vi "2_2_VisualAD_Inference(Camera).vi"() -> ()   [LabVIEW 2020]
uses:
  <vilib>/Ngene/DeepLTK Anomaly Detection Addon/Toolkit/API/Controls/NN_Paths.ctl
  <vilib>/Ngene/Deep Learning Toolkit/Toolkit/NN_Data/API/NN_Dims(C,H,W).ctl
  <vilib>/Ngene/Deep Learning Toolkit/Toolkit/NN_Network/Controls/NN_Device.ctl
  subVIs/Visualizer/Controls/Display_Options.ctl
  subVIs/Visualizer/Controls/ROI_Display_Options.ctl
  subVIs/Visualizer/Controls/Heatmap_Display_Options.ctl
  subVIs/Visualizer/Controls/ColorMap.ctl
  <vilib>/Ngene/DeepLTK Anomaly Detection Addon/Toolkit/API/Controls/MinMax.ctl
  subVIs/Visualizer/Controls/Report_Images_CFG.ctl
  subVIs/Camera/Controls/Camera_Settings.ctl
  <vilib>/Ngene/DeepLTK Anomaly Detection Addon/Toolkit/API/Controls/Crop_CFG.ctl
  <vilib>/Ngene/DeepLTK Anomaly Detection Addon/Toolkit/API/Controls/NNPC_Setup.ctl
  <vilib>/vision/driver/IMAQdx.llb/IMAQdx Camera Control Mode.ctl
  <vilib>/vision/driver/IMAQdx.llb/IMAQdx Buffer Number Mode.ctl
  <vilib>/Ngene/DeepLTK Anomaly Detection Addon/Toolkit/API/Controls/Feature_Scorer_Params.ctl
  <vilib>/Ngene/DeepLTK Anomaly Detection Addon/Toolkit/API/Controls/Gaussian_Blur.ctl
  <vilib>/Ngene/DeepLTK Anomaly Detection Addon/Toolkit/API/NNPC_Predict/NNPC_Predict(Single).vi
  <vilib>/Ngene/DeepLTK Anomaly Detection Addon/Toolkit/DeepLTK_Anomaly_Detection_Addon.lvlib
  <vilib>/ptbypt/NI_PtbyPt.lvlib
  <vilib>/vision/driver/NI_Vision_Acquisition_Software.lvlib
  <vilib>/Ngene/Deep Learning Toolkit/Toolkit/Deep_Learning_Toolkit_by_Ngene.lvlib
  <vilib>/Ngene/CuLab - GPU Accelerated Toolkit/Toolkit/CuLab.lvlib
panel:
  in  "Crop_CFG":T1={"Left"=0.0, "Top"=0.0, "Right"=1.0, "Bottom"=1.0}
  in  "Camera_Settings":T2={"Camera_Resolution"=10, "Focus"=0, "Exposure"=5, "Gain"=1, "WhiteB."=3000} {"WhiteB." min=2000 max=7500 step=1; "Gain" max=255 step=5; "Exposure" min=0 max=9 step=5; "Focus" step=5}
  in  "Rel Margin":sgl=0.02
  in  "Camera":refnum<k21>="cam0" caption="IMAQdx Session"
  out "Device Name":string="NVIDIA GeForce GTX 1650 Ti"
  in  "Display_Options":T3={"ROI_Options"={"Color"=16711713, "Width"=4, "Drawing Mode"=enum."Frame"}, "Heatmap_Options"={"ColorMap"=enum."Jet", "Alpha"=0.4, "Heatmap Range"={"Min"=25.0, "Max"=32.0}}, "Report_Images_CFG"={"Original Image"=TRUE, "Ground Truth"=TRUE, "HeatMap"=TRUE, "Mask"=TRUE, "Segmentation"=TRUE}} {"Heatmap_Options"."Heatmap Range"."Min" format="%#_5g"}
  in  "Trained_Model_Paths":T9={"CFG"=path "D:/Ngene/GitHub/deepltk_examples/3_Image_Processing/36_Anomaly_Detection/Models/NNPC_Cards_3ofHearts__25_10_21__19_21_13/NNPC_Cards_3ofHearts_25_10_21__19_21_13.cfg", "BIN"=path "D:/Ngene/GitHub/deepltk_examples/3_Image_Processing/36_Anomaly_Detection/Models/NNPC_Cards_3ofHearts__25_10_21__19_21_13/NNPC_Cards_3ofHearts_25_10_21__19_21_13.bin"}
  out "Anomaly?":bool=TRUE
  in  "Device":T10=enum."GPU"
  out "Dims_In":T11={"C"=3, "H"=120, "W"=160}
  out "Loop Time":dbl=0.02274215600000389 format="%.2ps"
  out "Preproc. Time":dbl=0.0010668470000018714 format="%.2ps"
  in  "Image_Thrshld":sgl=-1.0 format="%_5g"
  out "Pixel_Score(Max)":sgl=48.99041
  out "Img_Score":sgl=51.375824
  in  "Pixel_Thrshld":sgl=28.1 format="%_5g"
  out "Inference Time":dbl=0.010325968000006468 format="%.2ps"
  in  "Stop":bool
  out "Anomaly Detection Results":T12(plugin-control)
  # "Unsupervised \nVisual Anomaly Detection"
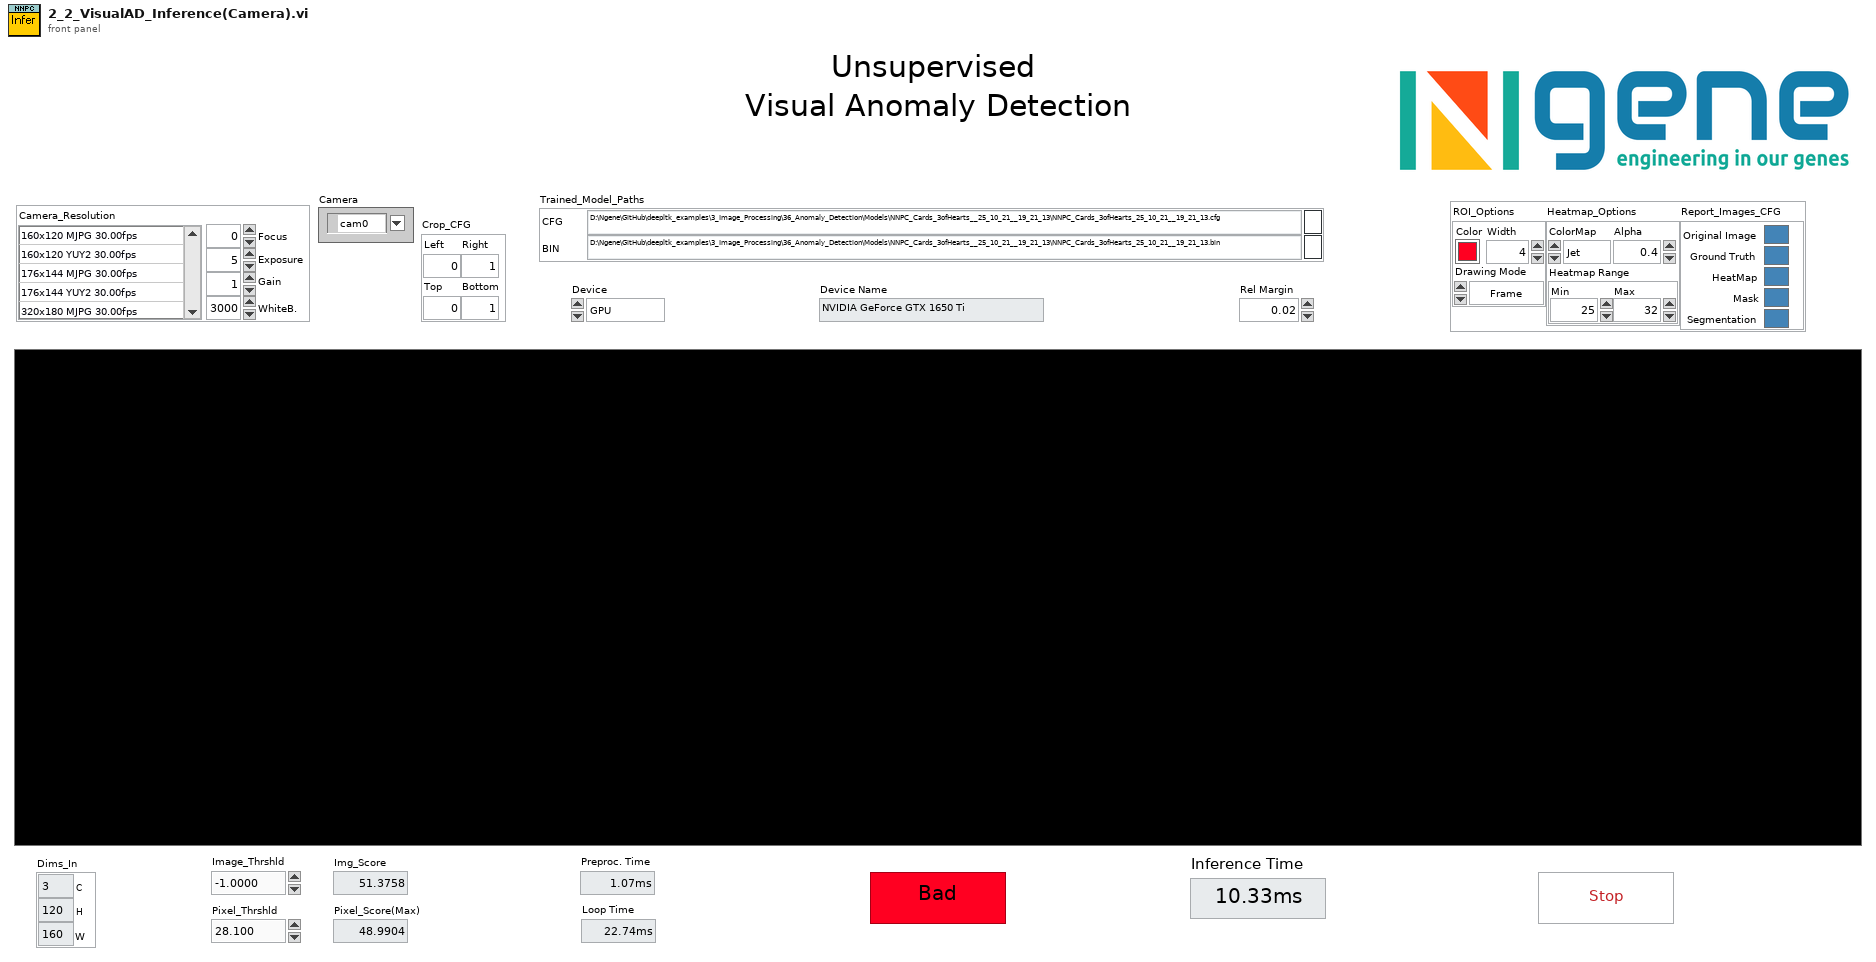
[diagram p1: front panel]
types:
  T1 = typedef "DeepLTK_Anomaly_Detection_Addon.lvlib/Crop_CFG.ctl" = cluster{"Left":sgl, "Top":sgl, "Right":sgl, "Bottom":sgl}
  T2 = typedef "Camera_Settings.ctl" = cluster{"Camera_Resolution":i32, "Focus":u8, "Exposure":i32, "Gain":u32, "WhiteB.":i32}
  T3 = typedef "Display_Options.ctl" = cluster{"ROI_Options":T4, "Heatmap_Options":T5, "Report_Images_CFG":T8}
  T4 = typedef "ROI_Display_Options.ctl" = cluster{"Color":u32, "Width":u32, "Drawing Mode":enum16{"Frame", "Fill"}}
  T5 = typedef "Heatmap_Display_Options.ctl" = cluster{"ColorMap":T6, "Alpha":sgl, "Heatmap Range":T7}
  T6 = typedef "ColorMap.ctl" = enum16{"Jet", "Perula", "Inferno", "Plasma", "Viridis"}
  T7 = typedef "DeepLTK_Anomaly_Detection_Addon.lvlib/MinMax.ctl" = cluster{"Min":sgl, "Max":sgl}
  T8 = typedef "Report_Images_CFG.ctl" = cluster{"Original Image":bool, "Ground Truth":bool, "HeatMap":bool, "Mask":bool, "Segmentation":bool}
  T9 = typedef "DeepLTK_Anomaly_Detection_Addon.lvlib/NN_Paths.ctl" = cluster{"CFG":path, "BIN":path}
  T10 = typedef "Deep_Learning_Toolkit_by_Ngene.lvlib/NN_Device.ctl" = enum16{"CPU", "GPU"}
  T11 = typedef "Deep_Learning_Toolkit_by_Ngene.lvlib/NN_Dims(C,H,W).ctl" = cluster{"C":i32, "H":i32, "W":i32}
  T12 = typedef "IMAQ Image.ctl" = refnum<image>
  T13 = typedef "NI_Vision_Acquisition_Software.lvlib/IMAQdx Camera Control Mode.ctl" = enum32{"Controller", "Listener"}
  T14 = typedef "Image Type" = u32
  T15 = typedef "DeepLTK_Anomaly_Detection_Addon.lvlib/NNPC_Setup.ctl" = cluster{"Input_Dims":T11, "mBatch":i32, "Device":T10, "GPU Id":i32}
  T16 = typedef "IMAQdx.ctl" = refnum<k21>
  T17 = typedef "DeepLTK_Anomaly_Detection_Addon.lvlib/NNPC_Evaluation_Results.ctl" = cluster{"Threshold(Image)":sgl, "Threshold(Pixel)":sgl, "Pixel_Range":cluster{"Min":sgl, "Max":sgl}}
  T18 = typedef "DeepLTK_Anomaly_Detection_Addon.lvlib/NNPC_PreProcessing_Options.ctl" = cluster{"DS_Name":string, "Input_Dims":T11, "Cropping":T1, "Interpolation Type":u32, "MultiStage_ReSample?":bool, "Dataset_Stats":T19}
  T19 = typedef "DeepLTK_Anomaly_Detection_Addon.lvlib/NNPC_DS_Stats.ctl" = cluster{"means":T20, "stds":T20}
  T20 = typedef "DeepLTK_Anomaly_Detection_Addon.lvlib/Image_Stats_RGB.ctl" = cluster{"R":sgl, "G":sgl, "B":sgl}
  T21 = typedef "DeepLTK_Anomaly_Detection_Addon.lvlib/NNPC_Instance.ctl" = cluster{"Name":string, "NN":T22, "MemBank_Data":T36}
  T22 = typedef "Deep_Learning_Toolkit_by_Ngene.lvlib/NN.ctl" = cluster{"Name":string, "No of Layers":i32, "mBatch":i32, "Layers":T23[], "Dimty":T24, "Dims_In":T11, "Dims_Out":T11, "Working_Dir":path, "Train?":bool, "Train_Params":T25, "LR_Update_Policy":T28, "Session Data":T30, "Ground_truth":T31, "NNg_hdls":T32, "NN_Device":T10, "GPU Id":i32, "Labels":string[], "Loss_Type":T33, "Loss_Cfg_Prms":variant, "NNG_WS":T34, "DryRun?":bool}
  T23 = typedef "Deep_Learning_Toolkit_by_Ngene.lvlib/NN_Layer_ref.ctl" = refnum<file>
  T24 = typedef "Deep_Learning_Toolkit_by_Ngene.lvlib/NN_In_Out_Dim-ty.ctl" = enum8{"In1D_Out1D", "In3D_Out1D", "In3D_Out3D", "In3D_OutBBox"}
  T25 = typedef "Deep_Learning_Toolkit_by_Ngene.lvlib/NN_Train_Params.ctl" = cluster{"Optimizer":T26, "Beta_1":sgl, "Beta_2":sgl, "Weight Decay(L1)":sgl, "Weight Decay(L2)":sgl, "Data_Sampling":T27}
  T26 = typedef "Deep_Learning_Toolkit_by_Ngene.lvlib/NN_Train_Optimizer.ctl" = enum16{"SGD", "Adam", "Adagrad", "Adadelta", "RMSProp", "Nesterov"}
  T27 = typedef "Deep_Learning_Toolkit_by_Ngene.lvlib/NN_Train_Data_Sampling.ctl" = enum16{"Random", "Sequential"}
  T28 = typedef "Deep_Learning_Toolkit_by_Ngene.lvlib/NN_LR_Policy_Cfg.ctl" = cluster{"Policy_Type":T29, "LR0":dbl, "k":sgl, "WarmUp_Policy":enum16{"Step", "Ramp"}, "WarmUp_Iter":i32, "WarmUp_Ratio":sgl}
  T29 = typedef "Deep_Learning_Toolkit_by_Ngene.lvlib/NN_LR_Policy_Type.ctl" = enum16{"Manual", "Step", "Exp", "1/t"}
  T30 = typedef "Deep_Learning_Toolkit_by_Ngene.lvlib/NN_Train_Session_Data.ctl" = cluster{"Epochs":sgl, "Tot_Iter":i32, "LR":sgl, "LR_iter":i32}
  T31 = typedef "Deep_Learning_Toolkit_by_Ngene.lvlib/NN_Ground_truth.ctl" = cluster{"Y":variant}
  T32 = typedef "Deep_Learning_Toolkit_by_Ngene.lvlib/nng_cuda_handles.ctl" = cluster{"cudnn":u64, "cublas":u64, "stream":u64, "curand":u64}
  T33 = typedef "Deep_Learning_Toolkit_by_Ngene.lvlib/NN_Loss_Type.ctl" = enum16{"None", "MSE", "CrossEntropy", "YOLO_v2", "YOLO_v4"}
  T34 = typedef "Deep_Learning_Toolkit_by_Ngene.lvlib/NNG_WS.ctl" = cluster{"NNG_WS_Mem":T35, "Max_WS_Size":i64}
  T35 = typedef "Deep_Learning_Toolkit_by_Ngene.lvlib/NNg_WS_Mem_DVR.ctl" = refnum<data-value>
  T36 = typedef "DeepLTK_Anomaly_Detection_Addon.lvlib/MemBank_and_Norm_Variants.ctl" = cluster{"MemBank":variant, "MemBank Norm":variant}
  T37 = typedef "DeepLTK_Anomaly_Detection_Addon.lvlib/Feature_Scorer_Params.ctl" = cluster{"Nearest_Neighbors":i32, "Calculate Anomaly Map":bool, "Gaussian_Blur":T38}
  T38 = typedef "DeepLTK_Anomaly_Detection_Addon.lvlib/Gaussian_Blur.ctl" = cluster{"Kernel_Size":i32, "Sigma":sgl}
  T39 = typedef "NI_Vision_Acquisition_Software.lvlib/IMAQdx Buffer Number Mode.ctl" = enum32{"Next", "Last", "Buffer Number", "Every", "Last New"}
  T40 = typedef "Anomaly_Detection_Results_Imgs.ctl" = cluster{"Image":T12, "Ground Truth":T12, "Predicted Heat Map":T12, "Predicted Mask":T12, "Segmentation":T12}
  T41 = typedef "CuLab.lvlib/Properties.ctl" = cluster{"Device ID":i32, "Name":string}
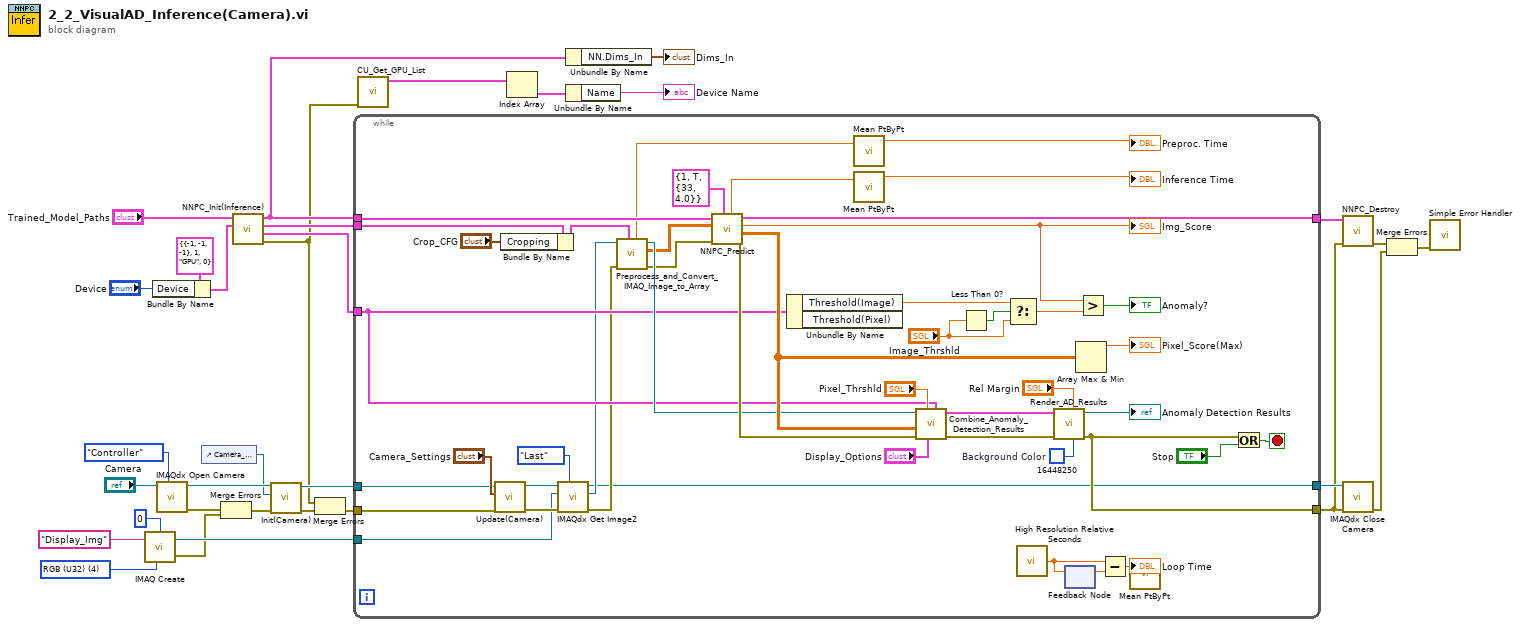
[diagram p0: block diagram]
diagram:
  w13 = T14 4 items=["Grayscale (U8)", "Grayscale (I16)", "Grayscale (SGL)", "Complex (CSG)", "RGB (U32)", "HSL (U32)", "RGB (U64)", "Grayscale (U16)"] ("Image Type")
  n1 = call "IMAQ Create"("Border Size"=0, "Image Name"="Display_Img", "Image Type"=w13) -> ("New Image"=w7:T12, "error out"=w4:errorcluster)  [unwired: 2 in]
  n2 = Bundle By Name(cluster=T15 {"Input_Dims"={"C"=-1, "H"=-1, "W"=-1}, "mBatch"=1, "Device"=enum."GPU", "GPU Id"=0} ("NNFE_CFG"), "Device"="Device") -> (w6:T15)
  n3 = call <vilib>:"IMAQdx Open Camera.vi"("Camera Control Mode"=IMAQdx_Camera_Control_Mode."Controller", "Session In"="Camera") -> ("error out"=w14:errorcluster, "Session Out"=w15:T16)  [unwired: 1 in, 7 out]
  n4 = control-ref of="Camera_Settings"() -> (w5:refnum<vi>)
  n5 = Merge Errors(w14, w4) -> (w10:errorcluster)
  n6 = call <vilib>:"NNPC_Init(Inference).vi"("NNPC_Setup"=w6, "NNPC_Paths"="Trained_Model_Paths") -> ("error out"=w2:errorcluster, "Evaluation_Results"=w28:T17, "PreProc_Options"=w29:T18, "NNPC_out"=w23:T21)  [unwired: 5 in, 1 out]
  n7 = call "Init(Camera).vi"("error in (no error)"=w10, "Camera_Settings_Ref"=w5, "Session in"=w15) -> ("error out"=w9:errorcluster, "Session out"=w8:T16)  [unwired: 7 in]
  n8 = Merge Errors(w2, w9) -> (w3:errorcluster)
  n9 = while {
    tunnel: w23 -> [w69]
    tunnel: [w64] -> w32
    tunnel: w29 -> [w56]
    tunnel: w28 -> [w51]
    tunnel: [w34] -> w27
    tunnel: [w50] -> w24
    tunnel: w3 -> [w42]
    tunnel: w8 -> [w33]
    tunnel: w7 -> [w41]
    stop <- w63 stop-if-true
    w62 = u32 16448250  # Background Color
    n10 = call "Update(Camera).vi"("error in (no error)"=w42, "Camera_Settings"="Camera_Settings", "Session in"=w33) -> ("error out"=w44:errorcluster, "Session out"=w43:T16)  [unwired: 7 in]
    n11 = Bundle By Name(cluster=w56, "Cropping"="Crop_CFG") -> (w36:T18)
    n12 = call <vilib>:"IMAQdx Get Image2.vi"("Buffer Number Mode (Next)"=IMAQdx_Buffer_Number_Mode."Last", "error in"=w44, "Image In"=w41, "Session In"=w43) -> ("error out"=w39:errorcluster, "Image Out"=w37:T12, "Session Out"=w34:T16)  [unwired: 4 in, 1 out]
    n13 = call "Preprocess_and_Convert_IMAQ_Image_to_Array.vi"("PreProcessing_Options"=w36, "error in (no error)"=w39, "Image In"=w37) -> ("error out"=w52:errorcluster, "Norm_Img_Out"=w38:sgl[][][], "Image_Out(PreProcessed)"=w53:T12, "dT_Preprocessing"=w54:dbl)  [unwired: 4 in, 1 out]
    n14 = call-poly <vilib>:"NNPC_Predict.vi"("Feature_Scorer_Params"=T37 {"Nearest_Neighbors"=1, "Calculate Anomaly Map"=TRUE, "Gaussian_Blur"={"Kernel_Size"=33, "Sigma"=4.0}}, "error in"=w52, "Image_in"=w38, "NNPC_in"=w69) -> ("error out"=w79:errorcluster, "Anomaly_Map"=w68:sgl[][], "Pred_Score"=w67:sgl, "NNPC_out"=w64:T21, "dT_Predict"=w61:dbl)  [unwired: 2 in, 1 out]
    "Img_Score" <- w67
    n15 = Unbundle By Name(w51) -> ("Threshold(Image)"=w60:sgl)  [unwired: 1 out]
    n16 = call <vilib>:"Mean PtByPt.vi"("x"=w54) -> ("mean"=→"Preproc. Time":dbl)  [unwired: 3 in, 1 out]
    n17 = call <vilib>:"Mean PtByPt.vi"("x"=w61) -> ("mean"=→"Inference Time":dbl)  [unwired: 3 in, 1 out]
    n18 = call "Combine_Anomaly_Detection_Results.vi"("Evaluation_Results"=w51, "Display_Options"="Display_Options", "Pixel Anomaly Thrshld"="Pixel_Thrshld", "error in"=w79, "Anomaly Map"=w68, "Orig Image In"=w53) -> ("error out"=w78:errorcluster, "Anomaly Detection Results"=w77:T40)  [unwired: 3 in, 1 out]
    n19 = Less Than 0?(x="Image_Thrshld") -> (x < 0?=w73:bool)
    n20 = Select(t=w60, s=w73, f="Image_Thrshld") -> (s? t:f=w71:sgl)
    n21 = call <vilib>:"High Resolution Relative Seconds.vi"() -> ("relative seconds"=w58:dbl)
    n22 = call "Render_AD_Results.vi"("Background Color"=w62, "Rel._Margin"="Rel Margin", "error in"=w78, "Anomaly Detection Rresults"=w77) -> ("error out"=w50:errorcluster, "Anomaly Detection Results"=→"Anomaly Detection Results":T12)  [unwired: 6 in]
    n23 = feedback #1() -> (w59:dbl)  [unwired: 1 in]
    n24 = feedback-in #1(w58) -> ()
    n25 = Array Max & Min(array=w68) -> (max value=→"Pixel_Score(Max)":sgl)  [unwired: 3 out]
    n26 = Greater?(x=w67, y=w71) -> (0:→"Anomaly?":bool)
    n27 = Subtract(x=w58, y=w59) -> (x-y=w57:dbl)
    n28 = call <vilib>:"Mean PtByPt.vi"("x"=w57) -> ("mean"=→"Loop Time":dbl)  [unwired: 3 in, 1 out]
    n29 = Or(x=w50, y="Stop") -> (x .or. y?=w63:bool)
  }
  n30 = call <vilib>:"CU_Get_GPU_List.vi"("error in (no error)"=w2) -> ("Devices"=w19:T41[])  [unwired: 9 in, 1 out]
  n31 = Index Array(array=w19) -> (element=w18:T41)  [unwired: 1 in]
  n32 = Unbundle By Name(w23) -> ("NN.Dims_In"=→"Dims_In":T11)
  n33 = Unbundle By Name(w18) -> ("Name"=→"Device Name":string)
  n34 = call <vilib>:"NNPC_Destroy.vi"("error in"=w24, "NNPC_in"=w32) -> ("error out"=w31:errorcluster)  [unwired: 9 in]
  n35 = call <vilib>:"IMAQdx Close Camera.vi"("error in"=w24, "Session In"=w27) -> ("error out"=w25:errorcluster)  [unwired: 9 out]
  n36 = Merge Errors(w31, w25) -> (w26:errorcluster)
  n37 = call <vilib>:"Simple Error Handler.vi"("error in (no error)"=w26) -> ()  [unwired: 4 in, 5 out]
